vi "PH_AWG-510.panel.vi"(0 "object ref":refnum<vi>, 5 "error in (no error)":errorcluster) -> (19 "error out":errorcluster)   [LabVIEW 2014, in "PH_AWG-510.lvlib"]
doc: "By this VI an ignitron can be monitored and switched. \n\n\"HEATING ON\" and \"WATER ON\" indicate the status (blue: bad tag value, no connection, or internal problems; lightgreen: on; red: off).\n\nThe button switches the electronic of the ignitron, \"SWITCH STATE\" indicates the switch status (blue: bad tag value, no connection, or internal problems; darkgreen: off; lightgreen: on).\n\n\"TRIGGER\" and \"TRIGGER PULSE\" indicate the status of the trigger (blue: bad tag value, no connection, or internal problems; darkgreen: off; lightgreen: on).\n\n\"on since\" indicates at which time the Ignition has been switched on.\n\n\"EXIT\" closes the front panel (GUI), while \"Delete Instance\" disconnects and removes the instance from the PCS.\n\nThis VI has no machine safety relevant logig: there is neither a check of internal conclict nor with other objects. Therefore it must be handled with care and should be operated by well educated operators only. It is forseen exclusively for direct operating and testing of the system. \n\nLicense Agreement for this software:\n\nCopyright (C)\nGesellschaft für Schwerionenforschung, GSI\nPlanckstr. 1\n64291 Darmstadt\nGermany\n\nContact: D.Beck@gsi.de \n\nThis program is free software; you can redistribute it and/or modify it under the terms of the GNU General Public License as published by the Free Software Foundation; either version 2 of the license, or (at your option) any later version.\n\nThis program is distributed in the hope that it will be useful, but WITHOUT ANYW ARRANTY; without even the implied warranty of MERCHANTABILITY or FITNESS FOR A PARTICULAR PURPOSE. See the GNU General License for more details (http://www.gnu.org).\n\nGesellschaft für Schwerionenforschung, GSI\nPlanckstr. 1, 64291 Darmstadt, Germany\nFor all questions and ideas contact: M.Richter@gsi.de, H.Brand@gsi.de or D.Beck@gsi.de.\nLast update: 18-DEC-2002"
uses:
  PH_AWG-510.lvlib
  PH_StatusHandler/PH_StatusHandler.GUI element.ctl
  PH_AWG-510.Instrument Information Dataset.ctl
  PH_AWG-510.Trigger Settings.ctl
  PH_AWG-510.Output Settings.ctl
  PH_Common/Names/PH_Names.File Types.ctl
  CSCore/CSObj/CSObj.lvlib
  PH_Common/PH_Common.lvlib
  CSCore/CSSystem/CSSystemLib/CSSystemLib.lvlib
  PH_PSDBWriter/PH_PSDBWriter.lvlib
  PH_Class/PH_Class.lvlib
  PH_StatusHandler/PH_StatusHandler.lvlib
panel:
  in  "Tab Control":enum32{"Trigger & Output", "Sets and Info"}(tab)
  in  "Configure Channel":bool
  in  "Channel Configuration":T1={"Activate Channel"=FALSE, "VPP (V)"=-1.0, "Clock (Hz)"=-1.0, "File Name (Device)"="", "#1"=0, "#2"=0, "#3"=0, "#4"=0, "#5"=0, "#6"=0, "#7"=0, "#8"=0, "#9"=0, "#10"=0, "#11"=0, "#12"=0, "#13"=0, "#14"=0, "#15"=0, "#16"=0, "#17"=0, "#18"=0, "#19"=0, "#20"=0, "Offset (V)"=-1.0} {"#20" max=1023 step=1 scale=0.0..1023.0; "#19" max=1023 step=1 scale=0.0..1023.0; "#18" max=1023 step=1 scale=0.0..1023.0; "#17" max=1023 step=1 scale=0.0..1023.0; "#16" max=1023 step=1 scale=0.0..1023.0; "#15" max=1023 step=1 scale=0.0..1023.0; "#14" max=1023 step=1 scale=0.0..1023.0; "#13" max=1023 step=1 scale=0.0..1023.0; "#12" max=1023 step=1 scale=0.0..1023.0; "#11" max=1023 step=1 scale=0.0..1023.0; "#10" max=1023 step=1 scale=0.0..1023.0; "#9" max=1023 step=1 scale=0.0..1023.0; "#8" max=1023 step=1 scale=0.0..1023.0; "#7" max=1023 step=1 scale=0.0..1023.0; "#6" max=1023 step=1 scale=0.0..1023.0; "#5" max=1023 step=1 scale=0.0..1023.0; "#4" max=1023 step=1 scale=0.0..1023.0; "#3" max=1023 step=1 scale=0.0..1023.0; "#2" max=1023 step=1 scale=0.0..1023.0; "#1" max=1023 step=1 scale=0.0..1023.0}
  in  "Trigger Settings":T2
  in  "Expert Mode":bool
  in  "Read Settings":bool
  in  "Save Settings":bool
  out "Waveform Settings File":path
  out "Instrument Information":T3
  in  "Lock Frontpanel":bool
  in  "Initialize":bool
  in  "Start Device":bool
  out "PSDB Status":u32(colorbox)=6618880 caption="PSDB"
  out "Status":T4 caption="State"
  in  "Delete":bool
  in  "Exit":bool
  # "PCS"
  # "3.40"
  # "Waveform Pattern"
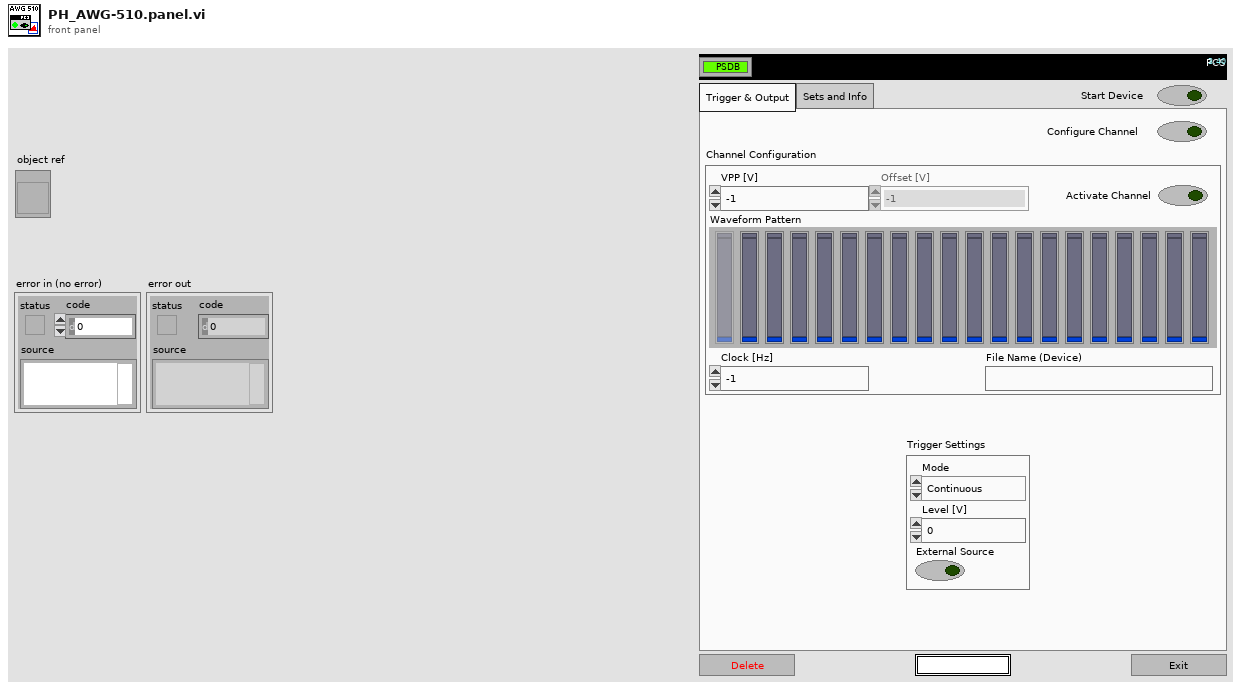
[diagram p1: front panel]
types:
  T1 = typedef "PH_AWG-510.lvlib/PH_AWG-510.Output Settings.ctl" = cluster{"Activate Channel":bool, "VPP (V)":dbl, "Clock (Hz)":dbl, "File Name (Device)":string, "#1":u16, "#2":u16, "#3":u16, "#4":u16, "#5":u16, "#6":u16, "#7":u16, "#8":u16, "#9":u16, "#10":u16, "#11":u16, "#12":u16, "#13":u16, "#14":u16, "#15":u16, "#16":u16, "#17":u16, "#18":u16, "#19":u16, "#20":u16, "Offset (V)":dbl}
  T2 = typedef "PH_AWG-510.lvlib/PH_AWG-510.Trigger Settings.ctl" = cluster{"Mode":enum16{"Continuous", "Triggered", "Gated", "Enhanced"}, "Level (V)":dbl, "External Source":bool}
  T3 = typedef "PH_AWG-510.lvlib/PH_AWG-510.Instrument Information Dataset.ctl" = cluster{"VISA resource name":refnum<visa-resource-name>, "Instrument Firmware Revision":string, "Manufacturer":string, "Model":string, "Serial Number":string, "Error Message":string, "Device Status":enum16{"stopped", "wating for trigger", "running", "Failure"}}
  T4 = typedef "PH_StatusHandler.lvlib/PH_StatusHandler.GUI element.ctl" = u16
  T5 = typedef "PH_Common.lvlib/PH_Names.File Types.ctl" = string
  T6 = typedef "PH_AWG-510.lvlib/PH_AWG-510.i attribute.ctl" = cluster{"GUI Refs":cluster{"Delete":refnum<vi>, "Trigger Settings":refnum<vi>, "Start Device":refnum<vi>, "Instrument Information":refnum<vi>, "Lock Frontpanel":refnum<vi>, "Waveform Pattern File":refnum<vi>, "Initialize":refnum<vi>, "Output Settings":refnum<vi>}, "Instrument Information":T3, "Initialized?":bool, "Current Settings":cluster{"Trigger":T2, "Output Settings":T1}, "Wanted Settings":cluster{"Trigger":T2, "Output Settings":T1}, "Device frontpanel locked?":bool, "Default File Path":path}
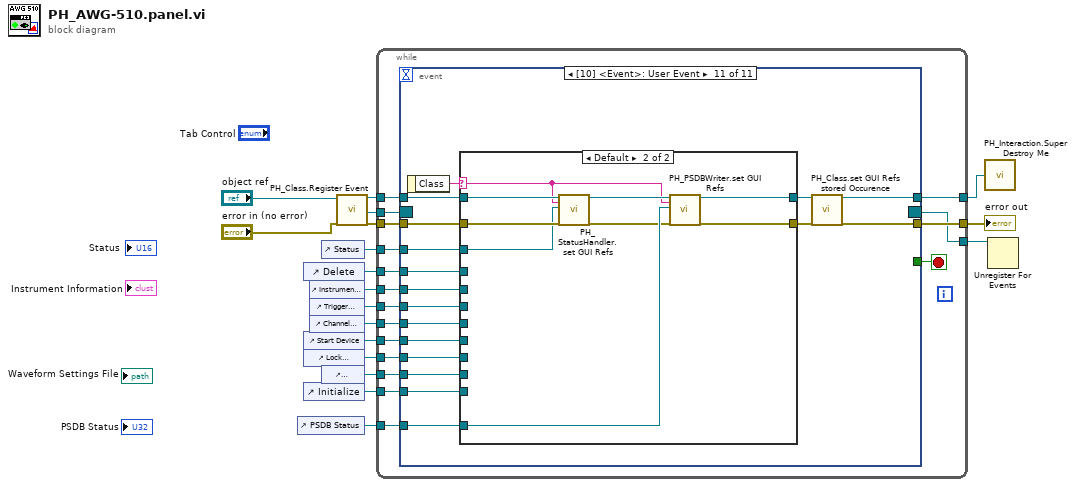
[diagram p0: block diagram]
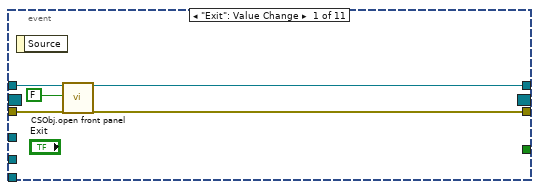
[diagram p2: hidden frame]
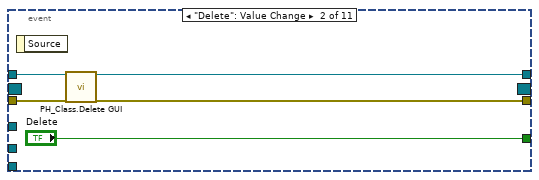
[diagram p3: hidden frame]
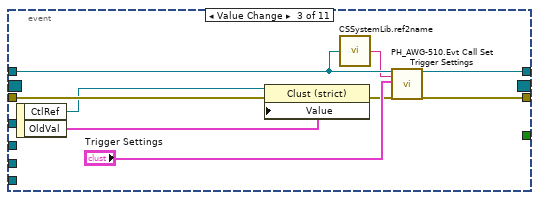
[diagram p4: hidden frame]
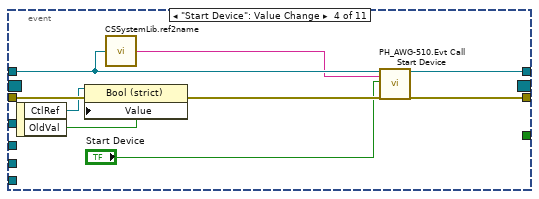
[diagram p5: hidden frame]
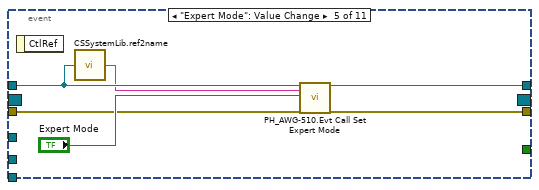
[diagram p6: hidden frame]
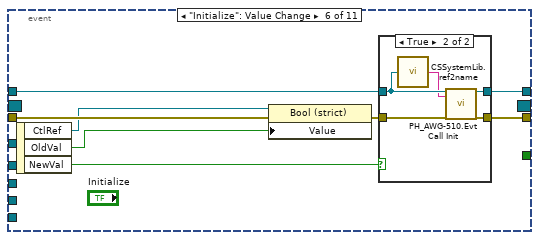
[diagram p7: hidden frame]
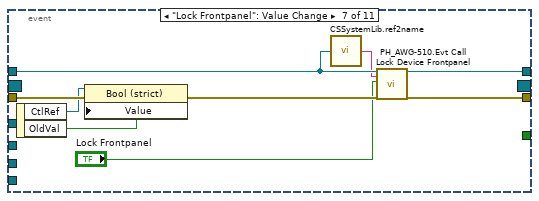
[diagram p9: hidden frame]
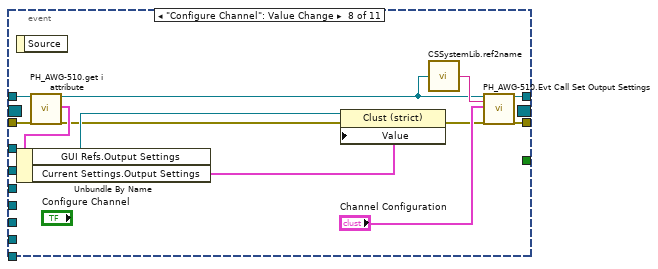
[diagram p10: hidden frame]
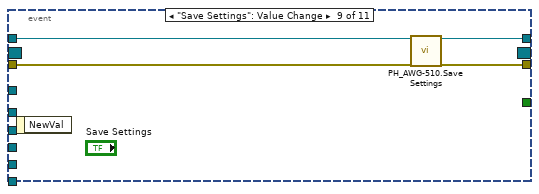
[diagram p11: hidden frame]
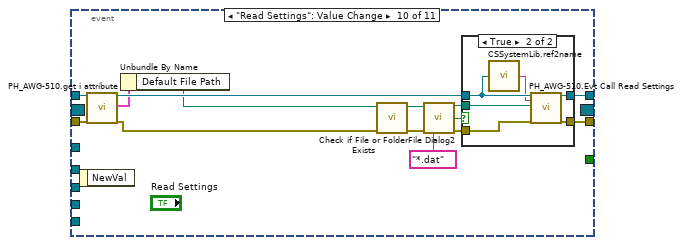
[diagram p12: hidden frame]
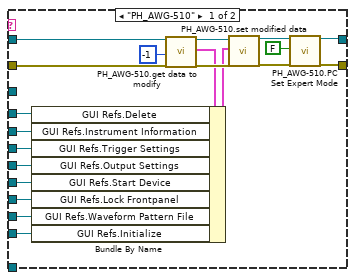
[diagram p14: hidden frame]
diagram:
  n1 = control-ref of="PSDB Status"() -> (w12:refnum<vi>)
  n2 = control-ref of="Delete"() -> (w9:refnum<vi>)
  n3 = control-ref of="Start Device"() -> (w4:refnum<vi>)
  n4 = control-ref of="Lock Frontpanel"() -> (w3:refnum<vi>)
  n5 = control-ref of="Initialize"() -> (w1:refnum<vi>)
  n6 = control-ref of="Instrument Information"() -> (w7:refnum<vi>)
  n7 = control-ref of="Trigger Settings"() -> (w6:refnum<vi>)
  n8 = control-ref of="Channel Configuration"() -> (w5:refnum<vi>)
  n9 = control-ref of="Status"() -> (w8:refnum<vi>)
  n10 = control-ref of="Waveform Settings File"() -> (w2:refnum<vi>)
  n11 = call "PH_Class.Register Event.vi"("i ref in"="object ref", "error in (no error)"="error in (no error)") -> ("i ref out"=w15:refnum<vi>, "Event Registration Refnum"=w14:refnum<event-registration>, "error out"=w16:errorcluster)  [unwired: 15 in]
  n12 = while {
    tunnel: w15 -> [w32]
    tunnel: [w31] -> w18
    tunnel: w16 -> [w34]
    tunnel: [w33] -> w17
    tunnel: w14 -> [w30]
    tunnel: [w29] -> w13
    tunnel: w12 -> [w28]
    tunnel: w9 -> [w27]
    tunnel: w8 -> [w26]
    tunnel: w7 -> [w25]
    tunnel: w6 -> [w24]
    tunnel: w5 -> [w23]
    tunnel: w4 -> [w22]
    tunnel: w3 -> [w21]
    tunnel: w2 -> [w20]
    tunnel: w1 -> [w19]
    stop <- w35 stop-if-true
    n13 = event shown="[10] <Event>: User Event" {
      selector: w30 -> [_ _ _ _ _ _ _ _ _ _ _]
      dyn-events: [_ _ _ _ _ _ _ _ _ _ _] -> w29
      timeout: _ -> [_ _ _ _ _ _ _ _ _ _ _]
      tunnel: [_ "Delete" _ _ _ _ _ _ _ _ _] -> w35
      tunnel: w32 -> [w40 w44 w51 w60 w67 w74 w90 w100 w107 w116 w148]
      tunnel: w34 -> [w38 w43 w53 w62 w64 w76 w92 w103 w106 w114 w147]
      tunnel: [w37 w42 w52 w61 w68 w75 w91 w104 w108 w122 w144] -> w33
      tunnel: [w36 w41 w54 w63 w69 w77 w93 w105 w109 w123 w142] -> w31
      tunnel: w28 -> [_ _ _ _ _ _ _ _ _ _ w145]
      tunnel: w27 -> [_ _ _ _ _ _ _ _ _ _ w140]
      tunnel: w26 -> [_ _ _ _ _ _ _ _ _ _ w139]
      tunnel: w25 -> [_ _ _ _ _ _ _ _ _ _ w138]
      tunnel: w24 -> [_ _ _ _ _ _ _ _ _ _ w137]
      tunnel: w23 -> [_ _ _ _ _ _ _ _ _ _ w136]
      tunnel: w22 -> [_ _ _ _ _ _ _ _ _ _ w135]
      tunnel: w21 -> [_ _ _ _ _ _ _ _ _ _ w134]
      tunnel: w20 -> [_ _ _ _ _ _ _ _ _ _ w133]
      tunnel: w19 -> [_ _ _ _ _ _ _ _ _ _ w132]
      event "Exit": Value Change {
        n14 = event-data() -> ()  [unwired: 1 in, 1 out]
        n15 = call "CSObj.open front panel.vi"("i ref in"=w40, "frontPanelOpen"=FALSE ("front panel open"), "error in (no error)"=w38) -> ("i ref out"=w36:refnum<vi>, "error out"=w37:errorcluster)  [unwired: 15 in]
      }
      event "Delete": Value Change {
        n16 = event-data() -> ()  [unwired: 1 in, 1 out]
        n17 = call "PH_Class.Delete GUI.vi"("VI in"=w44, "error in (no error)"=w43) -> ("VI out"=w41:refnum<vi>, "error out"=w42:errorcluster)  [unwired: 16 in]
      }
      event Value Change {
        n18 = event-data() -> ("CtlRef"=w47:refnum<vi>, "OldVal"=w46:T2)  [unwired: 1 in]
        n19 = property class="Clust (strict)"(reference=w47, error in=w53, "Value"=w46) -> (error out=w48:errorcluster)  [unwired: 1 out]
        n20 = call "CSSystemLib.ref2name.vi"("obj refnum"=w51) -> ("name"=w50:string)
        n21 = call "PH_AWG-510.Evt Call Set Trigger Settings.vi"("i ref in"=w51, "Instance"=w50, "Wanted Trigger Settings"="Trigger Settings", "error in"=w48) -> ("i ref out"=w54:refnum<vi>, "error out"=w52:errorcluster)  [unwired: 14 in]
      }
      event "Start Device": Value Change {
        n22 = event-data() -> ("CtlRef"=w57:refnum<vi>, "OldVal"=w56:bool)  [unwired: 1 in]
        n23 = property class="Bool (strict)"(reference=w57, error in=w62, "Value"=w56) -> (error out=w58:errorcluster)  [unwired: 1 out]
        n24 = call "CSSystemLib.ref2name.vi"("obj refnum"=w60) -> ("name"=w59:string)
        n25 = call "PH_AWG-510.Evt Call Start Device.vi"("i ref in"=w60, "Instance"=w59, "Start Device"="Start Device", "error in"=w58) -> ("i ref out"=w63:refnum<vi>, "error out"=w61:errorcluster)  [unwired: 14 in]
      }
      event "Expert Mode": Value Change {
        n26 = event-data() -> ()  [unwired: 1 in, 1 out]
        n27 = call "CSSystemLib.ref2name.vi"("obj refnum"=w67) -> ("name"=w66:string)
        n28 = call "PH_AWG-510.Evt Call Set Expert Mode.vi"("i ref in"=w67, "Instance"=w66, "Expert Mode"="Expert Mode", "error in"=w64) -> ("i ref out"=w69:refnum<vi>, "error out"=w68:errorcluster)  [unwired: 14 in]
      }
      event "Initialize": Value Change {
        n29 = event-data() -> ("CtlRef"=w72:refnum<vi>, "OldVal"=w71:bool, "NewVal"=w70:bool)  [unwired: 1 in]
        n30 = property class="Bool (strict)"(reference=w72, error in=w76, "Value"=w71) -> (error out=w73:errorcluster)  [unwired: 1 out]
        n31 = case shown="True" w70 {
          tunnel: [w79 w84] -> w77
          tunnel: [w78 w83] -> w75
          tunnel: w74 -> [w79 w82]
          tunnel: w73 -> [w78 w80]
          frame False {
          }
          frame True {
            n32 = call "CSSystemLib.ref2name.vi"("obj refnum"=w82) -> ("name"=w81:string)
            n33 = call "PH_AWG-510.Evt Call Init.vi"("i ref in"=w82, "Instance"=w81, "error in"=w80) -> ("i ref out"=w84:refnum<vi>, "error out"=w83:errorcluster)  [unwired: 15 in]
          }
        }
      }
      event "Lock Frontpanel": Value Change {
        n34 = event-data() -> ("CtlRef"=w87:refnum<vi>, "OldVal"=w86:bool)  [unwired: 1 in]
        n35 = property class="Bool (strict)"(reference=w87, error in=w92, "Value"=w86) -> (error out=w88:errorcluster)  [unwired: 1 out]
        n36 = call "CSSystemLib.ref2name.vi"("obj refnum"=w90) -> ("name"=w89:string)
        n37 = call "PH_AWG-510.Evt Call Lock Device Frontpanel.vi"("i ref in"=w90, "Instance"=w89, "Lock Device Frontpanel"="Lock Frontpanel", "error in"=w88) -> ("i ref out"=w93:refnum<vi>, "error out"=w91:errorcluster)  [unwired: 14 in]
      }
      event "Configure Channel": Value Change {
        n38 = event-data() -> ()  [unwired: 1 in, 1 out]
        n39 = call "PH_AWG-510.get i attribute.vi"("i ref in"=w100, "error in (no error)"=w103) -> ("i ref out"=w99:refnum<vi>, "i attribute"=w98:T6, "error out"=w96:errorcluster)  [unwired: 15 in]
        n40 = Unbundle By Name(w98) -> ("GUI Refs.Output Settings"=w97:refnum<vi>, "Current Settings.Output Settings"=w94:T1)
        n41 = property class="Clust (strict)"(reference=w97, error in=w96, "Value"=w94) -> (error out=w95:errorcluster)  [unwired: 1 out]
        n42 = call "CSSystemLib.ref2name.vi"("obj refnum"=w99) -> ("name"=w102:string)
        n43 = call "PH_AWG-510.Evt Call Set Output Settings.vi"("i ref in"=w99, "Instance"=w102, "Wanted Output Settings"="Channel Configuration", "error in"=w95) -> ("i ref out"=w105:refnum<vi>, "error out"=w104:errorcluster)  [unwired: 14 in]
      }
      event "Save Settings": Value Change {
        n44 = event-data() -> ()  [unwired: 1 in, 1 out]
        n45 = call "PH_AWG-510.Save Settings.vi"("VI in"=w107, "error in (no error)"=w106) -> ("VI out"=w109:refnum<vi>, "error out"=w108:errorcluster)  [unwired: 16 in]
      }
      event "Read Settings": Value Change {
        n46 = event-data() -> ()  [unwired: 1 in, 1 out]
        n47 = call "PH_AWG-510.get i attribute.vi"("i ref in"=w116, "error in (no error)"=w114) -> ("i ref out"=w115:refnum<vi>, "i attribute"=w112:T6, "error out"=w113:errorcluster)  [unwired: 15 in]
        n48 = Unbundle By Name(w112) -> ("Default File Path"=w111:path)
        n49 = call <vilib>:"Check if File or Folder Exists.vi"("error in (no error)"=w113, "path"=w111) -> ("error out"=w118:errorcluster, "dup path"=w117:path)  [unwired: 7 in, 1 out]
        n50 = call "File Dialog2"("start path"=w117, "error in"=w118, "pattern (all files)"=T5 "*.dat") -> ("selected path"=w120:path, "exists"=w119:bool, "error out"=w121:errorcluster)  [unwired: 9 in, 1 out]
        n51 = case shown="True" w119 {
          tunnel: [w125 w131] -> w123
          tunnel: [w124 w130] -> w122
          tunnel: w115 -> [w125 w129]
          tunnel: w121 -> [w124 w127]
          tunnel: w120 -> [_ w126]
          frame False {
          }
          frame True {
            n52 = call "CSSystemLib.ref2name.vi"("obj refnum"=w129) -> ("name"=w128:string)
            n53 = call "PH_AWG-510.Evt Call Read Settings.vi"("i ref in"=w129, "Instance"=w128, "Pattern File"=w126, "error in"=w127) -> ("i ref out"=w131:refnum<vi>, "error out"=w130:errorcluster)  [unwired: 14 in]
          }
        }
      }
      event User Event {
        n54 = event-data() -> ("Class"=w141:string)  [unwired: 1 in]
        n55 = case shown="Default" w141 {
          selector: w141 -> [_ w170]
          tunnel: w148 -> [w160 w172]
          tunnel: w147 -> [w158 w177]
          tunnel: [w157 w176] -> w146
          tunnel: w145 -> [_ w175]
          tunnel: [w159 w174] -> w143
          tunnel: w140 -> [w156 _]
          tunnel: w139 -> [_ w169]
          tunnel: w138 -> [w155 _]
          tunnel: w137 -> [w154 _]
          tunnel: w136 -> [w153 _]
          tunnel: w135 -> [w152 _]
          tunnel: w134 -> [w151 _]
          tunnel: w133 -> [w150 _]
          tunnel: w132 -> [w149 _]
          frame "PH_AWG-510" {
            n56 = call "PH_AWG-510.get data to modify.vi"("i ref in"=w160, "ms timeout (10000)"=-1, "error in (no error)"=w158) -> ("i ref out"=w168:refnum<vi>, "i attribute"=w166:T6, "error out"=w167:errorcluster)  [unwired: 13 in, 1 out]
            n57 = Bundle By Name(cluster=w166, "GUI Refs.Delete"=w156, "GUI Refs.Instrument Information"=w155, "GUI Refs.Trigger Settings"=w154, "GUI Refs.Output Settings"=w153, "GUI Refs.Start Device"=w152, "GUI Refs.Lock Frontpanel"=w151, "GUI Refs.Waveform Pattern File"=w150, "GUI Refs.Initialize"=w149) -> (w165:T6)
            n58 = call "PH_AWG-510.set modified data.vi"("i ref in"=w168, "i attribute"=w165, "error in (no error)"=w167) -> ("i ref out"=w162:refnum<vi>, "error out"=w161:errorcluster)  [unwired: 15 in]
            n59 = call "PH_AWG-510.PC Set Expert Mode.vi"("VI in"=w162, "Expert Mode"=FALSE, "error in (no error)"=w161) -> ("VI out"=w159:refnum<vi>, "error out"=w157:errorcluster)  [unwired: 15 in]
          }
          frame Default {
            n60 = call "PH_StatusHandler.set GUI Refs.vi"("i ref in"=w172, "Class"=w170, "GUI Ref"=w169, "error in (no error)"=w177) -> ("i ref out"=w171:refnum<vi>, "error out"=w173:errorcluster)  [unwired: 14 in]
            n61 = call "PH_PSDBWriter.set GUI Refs.vi"("i ref in"=w171, "Class"=w170, "Ref PSDB Status"=w175, "error in"=w173) -> ("i ref out"=w174:refnum<vi>, "error out"=w176:errorcluster)  [unwired: 14 in]
          }
        }
        n62 = call "PH_Class.set GUI Refs stored Occurence.vi"("i ref in"=w143, "error in (no error)"=w146) -> ("i ref out"=w142:refnum<vi>, "error out"=w144:errorcluster)  [unwired: 16 in]
      }
    }
  }
  "error out" <- w17
  n63 = call "PH_Interaction.Super Destroy Me.vi"("i ref out"=w18) -> ()
  n64 = Unregister For Events(event registration refnum=w13) -> ()  [unwired: 1 in, 1 out]
